vi "Caller VI.vi"() -> ()   [LabVIEW 2025]
uses:
  CLD3 FGV Mode.ctl
panel:
  in  "Timer Mode":T1=enum."Read Time"
  out "Has Time Elapsed":bool
  in  "stop":bool
  out "Elapsed Time (s.ss)":dbl
  out "Error Out":errorcluster
  in  "Error In":errorcluster
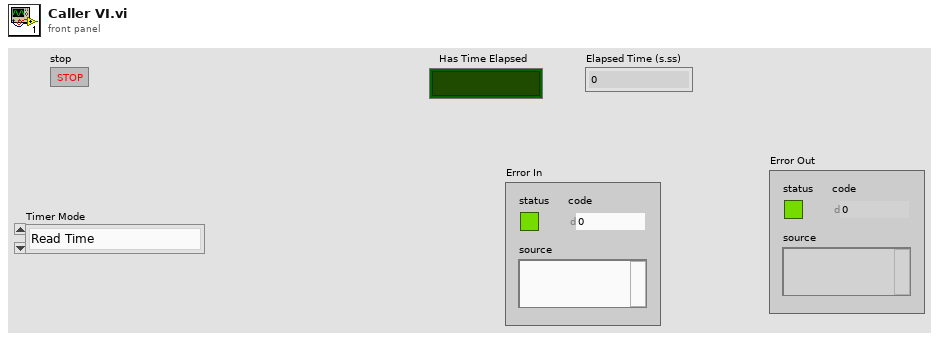
[diagram p1: front panel]
types:
  T1 = typedef "CLD3 FGV Mode.ctl" = enum16{"Start Timer", "Read Time", "Pause", "Resume"}
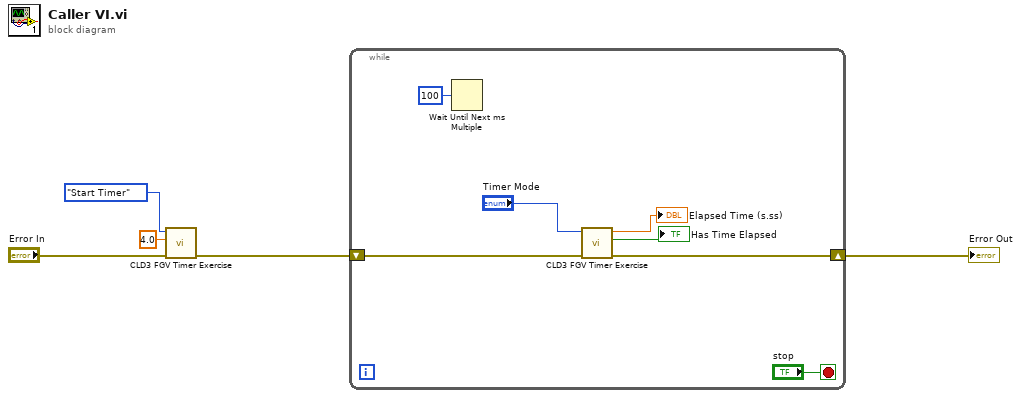
[diagram p0: block diagram]
diagram:
  n1 = call "CLD3 FGV Timer Exercise.vi"("Error In"="Error In", "Time Target (s)"=4.0, "Timer Mode"=CLD3_FGV_Mode."Start Timer") -> ("Error Out"=w4:errorcluster)  [unwired: 6 in, 2 out]
  n2 = while {
    shift-right: [w10] -> w1
    shift-left: w4 -> [w12]
    stop <- "stop" stop-if-true
    n3 = Wait Until Next ms Multiple(millisecond multiple=u32 100) -> ()  [unwired: 1 out]
    n4 = call "CLD3 FGV Timer Exercise.vi"("Error In"=w12, "Timer Mode"="Timer Mode") -> ("Error Out"=w10:errorcluster, "Has Time Elapsed"=→"Has Time Elapsed":bool, "Elapsed Time (s.ss)"=→"Elapsed Time (s.ss)":dbl)  [unwired: 7 in]
  }
  "Error Out" <- w1
